vi "Launcher.vi"() -> ()   [LabVIEW 2022 SP3]
uses:
  Axis Objects/iMotion Controller/iMotion Controller.lvclass
  148c7043-a0e6-40f1-af8e-846f2eb82a0e.vi
  58421ff6-31ce-4a07-9265-554c6ce1187d.vi
  148c7043-a0e6-40f1-af8e-846f2eb82a0e.vi/a9559f68-c05e-40f8-8ef8-fb73dbc3861a.vi
  58421ff6-31ce-4a07-9265-554c6ce1187d.vi/a9559f68-c05e-40f8-8ef8-fb73dbc3861a.vi
  XY Stage Controller/XY Stage Controller.lvclass
  C:/Stage-Work/MAS/2-Axis Stage API/2-Axis Stage API.lvclass
  <vilib>/Utility/LVClass/Get LV Class Default Value.vi
  Framework/Read Configs/Read Configs Sections.lvlib
panel:
  out "error out":errorcluster
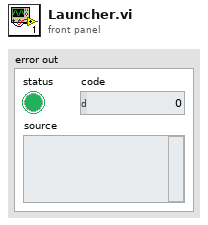
[diagram p1: front panel]
types:
  T1 = typedef "Read Configs Sections.lvlib/Section Data.ctl" = cluster{"Componets":string[], "Path":path, "Section":string}
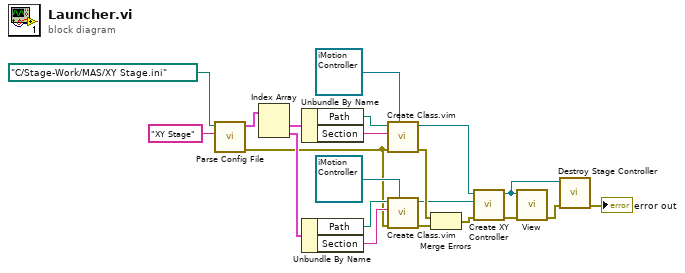
[diagram p0: block diagram]
diagram:
  n1 = call "Parse Config File.vi"("Section"="XY Stage", "Config Path"=path "C:/Stage-Work/MAS/XY Stage.ini") -> ("error out"=w8:errorcluster, "Array"=w21:T1[])  [unwired: 8 in]
  n2 = Index Array(array=w21) -> (element #1=w20:T1, element #2=w16:T1)  [unwired: 2 in]
  n3 = Unbundle By Name(w20) -> ("Path"=w18:path, "Section"=w17:string)
  n4 = Unbundle By Name(w16) -> ("Path"=w15:path, "Section"=w14:string)
  n5 = call "Create Class.vim"("Dynamic Load.lvclass"=refnum<class "iMotion Controller.lvclass"> refnum ("iMotion Controller.lvclass"), "error in (no error)"=w8, "Section"=w17, "Path"=w18) -> ("error out"=w10:errorcluster, "Dynamic Load out"=w5:refnum<class "iMotion Controller.lvclass">)  [unwired: 6 in]
  n6 = call "Create Class.vim"("Dynamic Load.lvclass"=refnum<class "iMotion Controller.lvclass"> refnum ("iMotion Controller.lvclass"), "error in (no error)"=w8, "Section"=w14, "Path"=w15) -> ("error out"=w9:errorcluster, "Dynamic Load out"=w4:refnum<class "iMotion Controller.lvclass">)  [unwired: 6 in]
  n7 = Merge Errors(w10, w9) -> (w2:errorcluster)
  n8 = call "Create XY Controller.vi"("error in (no error)"=w2, "Y-Axis"=w4, "X-Axis"=w5) -> ("error out"=w1:errorcluster, "XY Stage Controller out"=w3:refnum<class "XY Stage Controller.lvclass">)  [unwired: 7 in]
  n9 = call "View.vi"("error out"=w1, "2-Axis Stage"=w3) -> ("error out 2"=w6:errorcluster)  [unwired: 9 in]
  n10 = call "Destroy Stage Controller.vi"("error in (no error)"=w6, "XY Stage Controller in"=w3) -> ("error out"=→"error out":errorcluster)  [unwired: 8 in, 1 out]
